vi "LvMPDC_CMD_lsinfo.vi"(6 "timeout_ms":i32=25000, 8 "error in (no error)":errorcluster, 9 "ReadBytes":i32=1024, 10 "filepath":path, 11 "Connect ID":refnum<k5>) -> (0 "error out":errorcluster, 1 "file info[]":T2(array[cluster]) {"MusicInfo"."time" format="%<%H:%M:%S%3u>t"}, 2 "folder info[]":T2(array[cluster]) {"MusicInfo"."time" format="%<%H:%M:%S%3u>t"}, 3 "Connect ID out":refnum<k5>)   [LabVIEW 2012]
uses:
  LvMPDC_Typdef_MusicInfo.ctl
panel:
  # "LvMPDC:: CMD lsinfo"
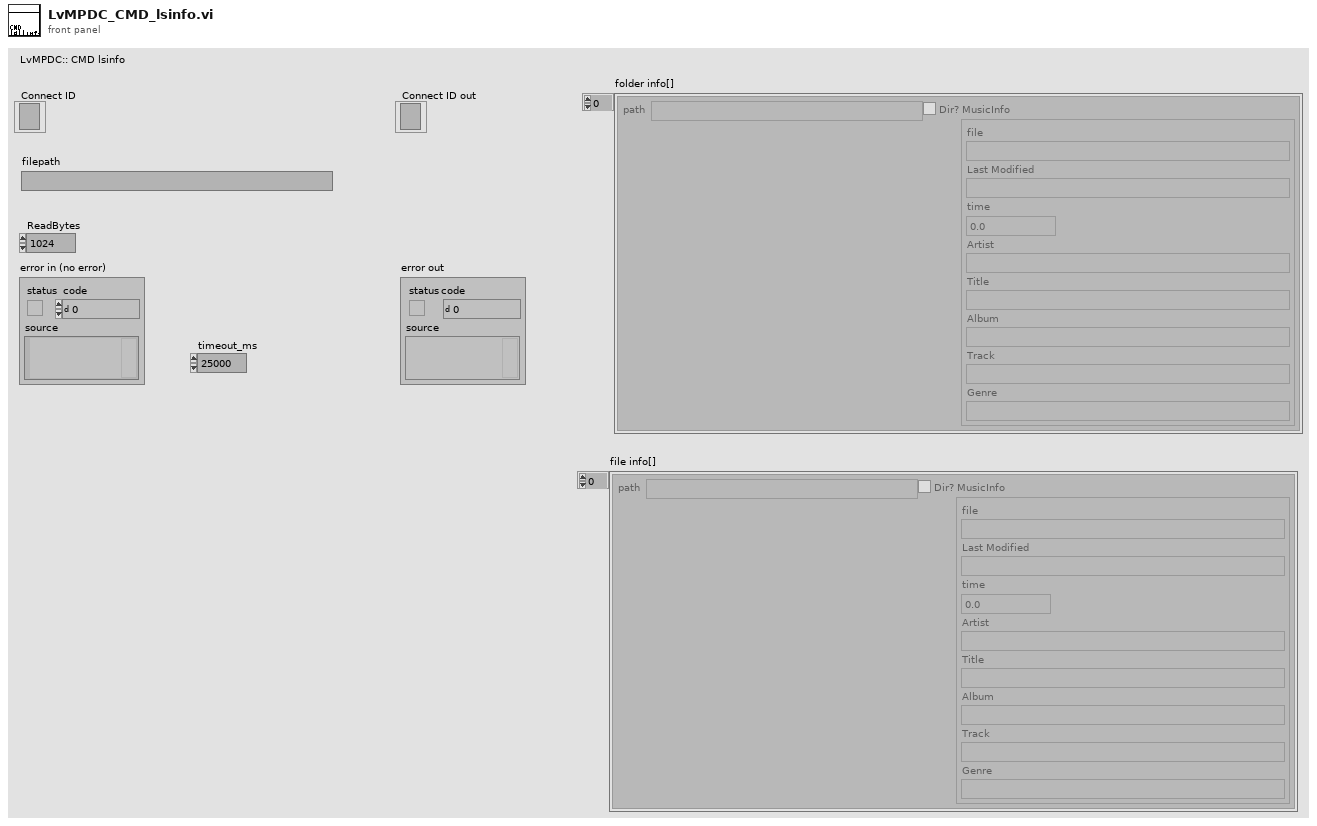
[diagram p1: front panel]
types:
  T1 = typedef "LvMPDC_Typdef_MusicInfo.ctl" = cluster{"file":string, "Last Modified":string, "time":dbl, "Artist":string, "Title":string, "Album":string, "Track":string, "Genre":string}
  T2 = cluster{"path":path, "Dir?":bool, "MusicInfo":T1}[]
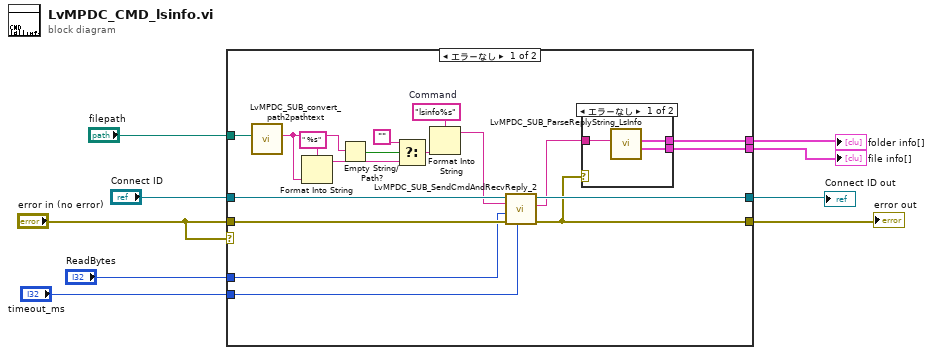
[diagram p0: block diagram]
diagram:
  n1 = case shown="エラーなし" "error in (no error)" {
    tunnel: "Connect ID" -> [w26 w32]
    tunnel: "error in (no error)" -> [w27 w31]
    tunnel: [w25 w32] -> w8
    tunnel: [w22 w31] -> w7
    tunnel: "timeout_ms" -> [w23 _]
    tunnel: "ReadBytes" -> [w24 _]
    tunnel: "filepath" -> [w20 _]
    tunnel: [w11 _] -> w2
    tunnel: [w10 _] -> w1
    frame No Error {
      w12 = "lsinfo%s"  # Command
      n2 = call "LvMPDC_SUB_convert_path2pathtext.vi"("path"=w20) -> ("pathtext"=w16:string)  [unwired: 10 in]
      n3 = Format Into String(format string=" %s" ("形式文字列"), w16) -> (resulting string=w13:string)  [unwired: 2 in, 1 out]
      n4 = Empty String/Path?(string/path=w16) -> (empty?=w15:bool)
      n5 = Select(t="", s=w15, f=w13) -> (s? t:f=w17:string)
      n6 = Format Into String(format string=w12, w17) -> (resulting string=w19:string)  [unwired: 2 in, 1 out]
      n7 = call "LvMPDC_SUB_SendCmdAndRecvReply_2.vi"("timeout_ms"=w23, "error in (no error)"=w27, "ReadBytes"=w24, "Command"=w19, "Connect ID"=w26) -> ("error out"=w22:errorcluster, "Reply"=w21:string, "Connect ID out"=w25:refnum<k5>)  [unwired: 4 in]
      n8 = case shown="エラーなし" w22 {
        tunnel: w21 -> [w30 _]
        tunnel: [w29 _] -> w11
        tunnel: [w28 _] -> w10
        frame No Error {
          n9 = call "LvMPDC_SUB_ParseReplyString_LsInfo.vi"("string"=w30) -> ("file info[]"=w28:T2, "folder info[]"=w29:T2)  [unwired: 9 in]
        }
        frame Error {
        }
      }
    }
    frame Error {
    }
  }
  "Connect ID out" <- w8
  "error out" <- w7
  "file info[]" <- w1
  "folder info[]" <- w2
